vi "EV Loop Control.vi"(0 "Run Step Inputs":T1={"Data in"=[], "Results in"=[], "Seq Setup in"="", "Step name"="", "Hardware in"="", "Calibration in"="", "Step # in sequence"=0, "Display step?(f)"=TRUE, "Generate names only"=FALSE, "Waveforms in"=[], "Memory List Grouping info"=[]} {"Waveforms in"."Y dB ref" format="%.1f"; "Waveforms in"."Y axis" items=["dB", "Lin", "Pwr"]; "Waveforms in"."Y data" items=["dB", "Lin", "Pwr"]; "Waveforms in"."X data" items=["dB", "Lin", "Pwr"]; "Data in"."Z data" items=["dB", "Lin", "Pwr"]; "Data in"."X data" items=["dB", "Lin", "Pwr"]; "Data in"."Y data" items=["dB", "Lin", "Pwr"]; "Data in"."Z dB ref" format="%.1f"; "Data in"."Z axis" items=["Log", "Lin"]; "Data in"."X dB ref" format="%.1f"; "Data in"."X axis" items=["Log", "Lin"]; "Data in"."Y axis" items=["Log", "Lin"]; "Data in"."Y dB ref" format="%.1f"; "Data in"."Curve"."z" format="%.2f"; "Data in"."Curve"."y" format="%.2f"; "Data in"."Curve"."x" format="%.2f"; "Results in"."Unit type" items=["dB", "Lin", "Pwr"]; "Results in"."Margin" format="%.2f"}, 11 "error in (no error)":errorcluster) -> (6 "Data out":T2 {"Z data" items=["dB", "Lin", "Pwr"]; "X data" items=["dB", "Lin", "Pwr"]; "Y data" items=["dB", "Lin", "Pwr"]; "Z dB ref" format="%.1f"; "Z axis" items=["Log", "Lin"]; "X dB ref" format="%.1f"; "X axis" items=["Log", "Lin"]; "Y axis" items=["Log", "Lin"]; "Y dB ref" format="%.1f"; "Curve"."z" format="%.2f"; "Curve"."y" format="%.2f"; "Curve"."x" format="%.2f"}, 8 "Results out":T5 {"Unit type" items=["dB", "Lin", "Pwr"]; "Margin" format="%.2f"}, 10 "Waveforms out":T7 {"Y dB ref" format="%.1f"; "Y axis" items=["dB", "Lin", "Pwr"]; "Y data" items=["dB", "Lin", "Pwr"]; "X data" items=["dB", "Lin", "Pwr"]}, 15 "error out":errorcluster)   [LabVIEW 2014]
uses:
  custom and SC Run Seq Sub VIs (x64).llb/data array.ctl
  custom and SC Run Seq Sub VIs (x64).llb/data cluster.ctl
  custom and SC Run Seq Sub VIs (x64).llb/Axis Unit Type.ctl
  custom and SC Run Seq Sub VIs (x64).llb/result array.ctl
  custom and SC Run Seq Sub VIs (x64).llb/result cluster.ctl
  custom and SC Run Seq Sub VIs (x64).llb/waveform array.ctl
  custom and SC Run Seq Sub VIs (x64).llb/waveform cluster.ctl
  custom and SC Run Seq Sub VIs (x64).llb/Run Step Inputs.ctl
  custom and SC Run Seq Sub VIs (x64).llb/Memory List Grouping.ctl
  custom and SC Run Seq Sub VIs (x64).llb/Memory List Grouping - Item Type.ctl
  custom and SC Run Seq Sub VIs (x64).llb/window stack manager Functions.ctl
panel:
  out "mp curve":cluster{"x":dbl, "y":dbl, "z":dbl}[](array[cluster])
  out "inc curve":cluster{"x":dbl, "y":dbl, "z":dbl}[](array[cluster])
  out "x > 0?":bool
  out "size(s)":i32
  out "Numeric":dbl
  out "y":dbl
  out "x":dbl
  # "NOTE:  These controls and indicators must stay here, but you can Hide them if you wish.  These are wired as the standard input/output connector pane for step run VIs."
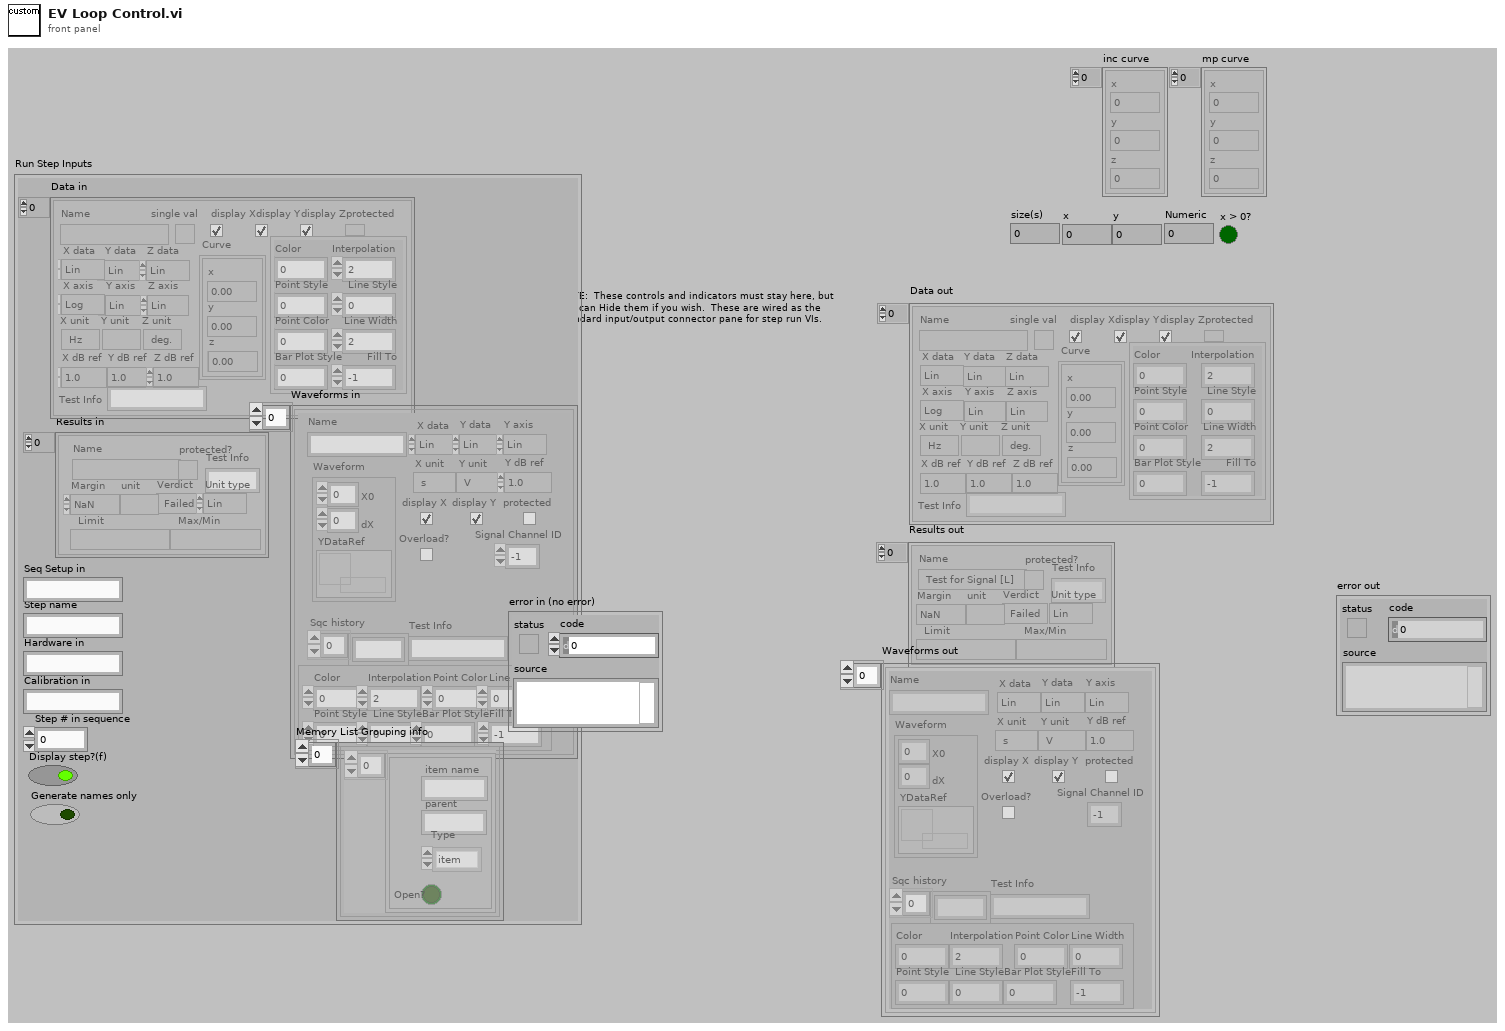
[diagram p1: front panel]
types:
  T1 = typedef "Run Step Inputs.ctl" = cluster{"Data in":T2, "Results in":T5, "Seq Setup in":string, "Step name":string, "Hardware in":string, "Calibration in":string, "Step # in sequence":i32, "Display step?(f)":bool, "Generate names only":bool, "Waveforms in":T7, "Memory List Grouping info":cluster{T9[]}[]}
  T2 = typedef "data array.ctl" = T3[]
  T3 = typedef "data cluster.ctl" = cluster{"Name":string, "Curve":cluster{"x":dbl, "y":dbl, "z":dbl}[], "X data":T4, "Y data":T4, "Z data":T4, "X axis":u16, "Y axis":u16, "Z axis":u16, "X unit":string, "Y unit":string, "Z unit":string, "X dB ref":dbl, "Y dB ref":dbl, "Z dB ref":dbl, "single val":bool, "protected":bool, "display X":bool, "display Y":bool, "display Z":bool, "Plot Settings":cluster{"Color":u32, "Interpolation":u8, "Point Style":u8, "Line Style":u8, "Point Color":u32, "Line Width":u8, "Bar Plot Style":u8, "Fill To":i16}, "Test Info":string}
  T4 = typedef "Axis Unit Type.ctl" = u16
  T5 = typedef "result array.ctl" = T6[]
  T6 = typedef "result cluster.ctl" = cluster{"Name":string, "Margin":dbl, "unit":string, "Verdict":bool, "Limit":string, "Max/Min":string, "protected?":bool, "Test Info":string, "Unit type":T4}
  T7 = typedef "waveform array.ctl" = T8[]
  T8 = typedef "waveform cluster.ctl" = cluster{"Name":string, "Waveform":cluster{"X0":dbl, "dX":dbl, "YDataRef":refnum<data-value>}, "X data":T4, "Y data":T4, "Y axis":T4, "X unit":string, "Y unit":string, "Y dB ref":dbl, "display Y":bool, "display X":bool, "Overload?":bool, "protected":bool, "Sqc history":string[], "Signal Channel ID":i32, "Plot Settings":cluster{"Color":u32, "Interpolation":u8, "Point Style":u8, "Line Style":u8, "Point Color":u32, "Line Width":u8, "Bar Plot Style":u8, "Fill To":i16}, "Test Info":string}
  T9 = typedef "Memory List Grouping.ctl" = cluster{"item name":string, "parent":string, "Open?":bool, "Type":T10}
  T10 = typedef "Memory List Grouping - Item Type.ctl" = enum16{"item", "custom group", "auto group", "protected group"}
  T11 = typedef "window stack manager Functions.ctl" = enum16{"Init", "add", "remove", "run", "clear", "vi stopped offset", "minimize all", "restore all", "autoadd", "Hourglass On", "Hourglass Off"}
  T12 = typedef "seq step setup.ctl" = cluster{"Input Signal Channels":i32[], "Output Signal Channels":i32[], "Curves selected":string[][], "Curves generated":string[], "Step setup flat":string, "Trigger Signal Channel":i32, "Curves Generated Assumptions":cluster{"seq-setup in":string, "Relevant subset of mem list Grouping":cluster{T9[]}[]}}
  T13 = cluster{"Curve[0]":cluster{"x":dbl, "y":dbl, "z":dbl}, "Curve[1]":cluster{"x":dbl, "y":dbl, "z":dbl}, "Curve[2]":cluster{"x":dbl, "y":dbl, "z":dbl}, "Curve[3]":cluster{"x":dbl, "y":dbl, "z":dbl}, "Curve[4]":cluster{"x":dbl, "y":dbl, "z":dbl}, "Curve[5]":cluster{"x":dbl, "y":dbl, "z":dbl}, "Curve[6]":cluster{"x":dbl, "y":dbl, "z":dbl}, "Curve[7]":cluster{"x":dbl, "y":dbl, "z":dbl}, "Curve[8]":cluster{"x":dbl, "y":dbl, "z":dbl}}
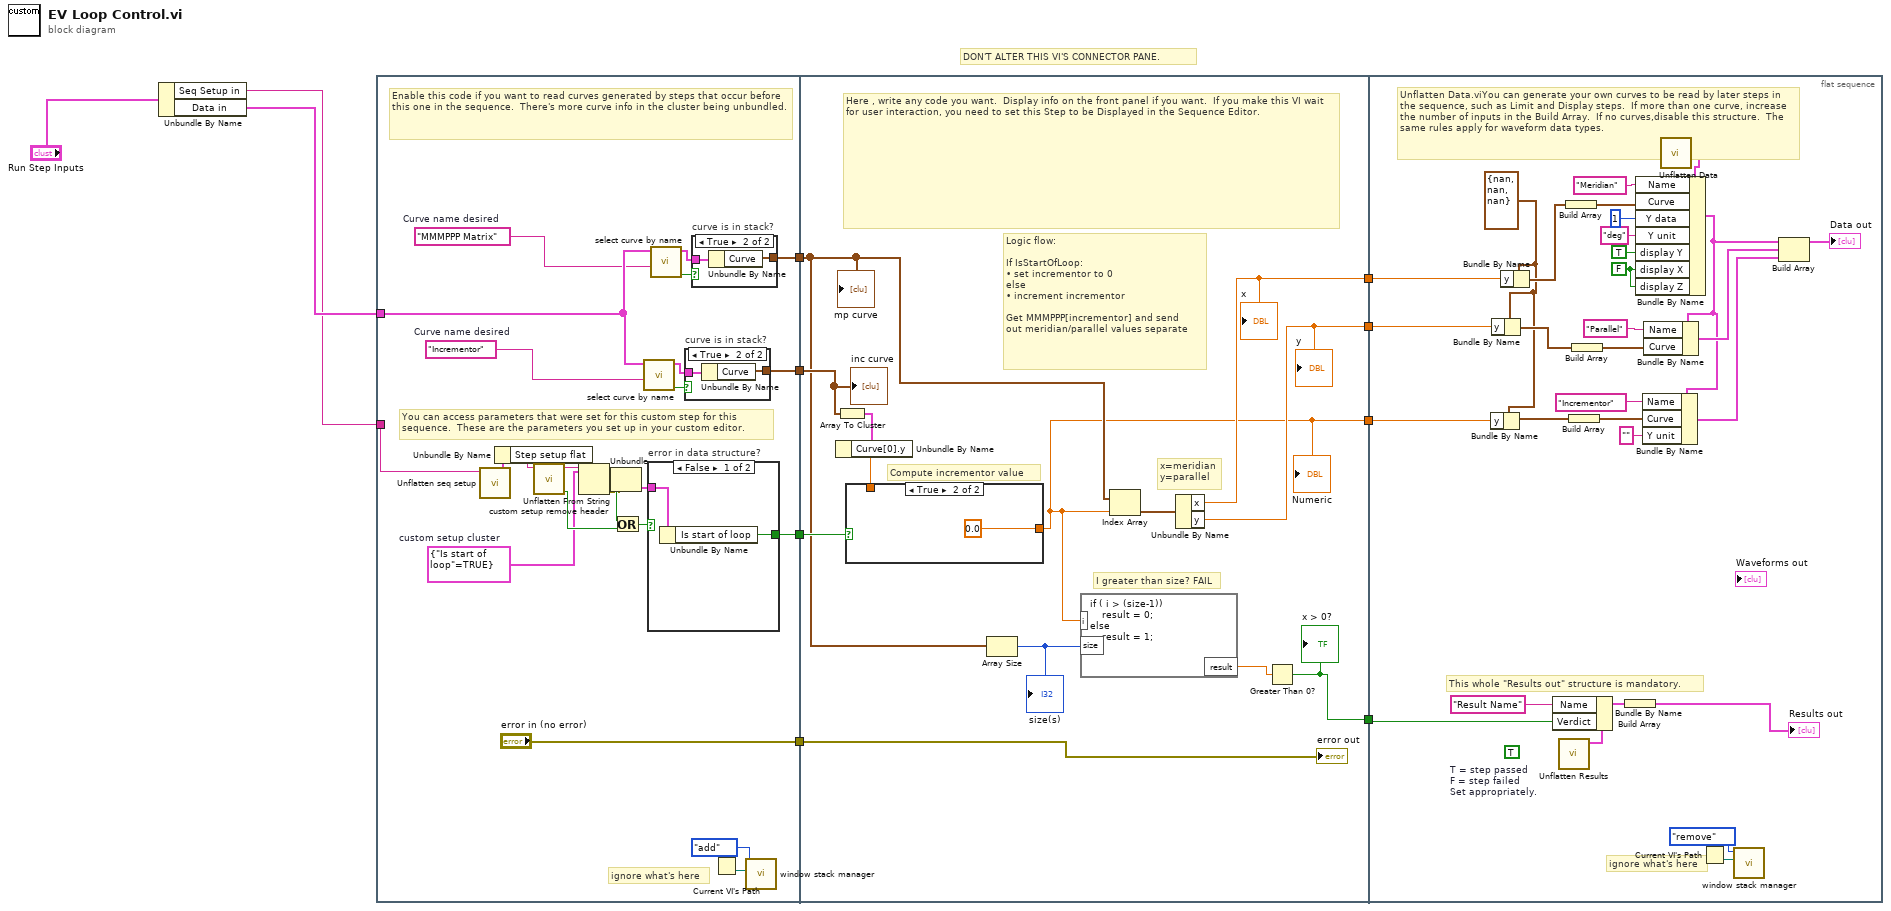
[diagram p0: block diagram]
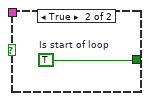
[diagram p4: hidden frame]
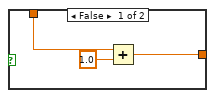
[diagram p5: hidden frame]
diagram:
  # "DON'T ALTER THIS VI'S CONNECTOR PANE."
  n1 = Unbundle By Name("Run Step Inputs") -> ("Seq Setup in"=w9:string, "Data in"=w10:T2)
  n2 = flat-sequence {
    tunnel: w10 -> [w15]
    tunnel: w9 -> [w25]
    tunnel: ["error in (no error)"] -> w8
    tunnel: [w19] -> w7
    tunnel: [w16] -> w6
    tunnel: [w14] -> w4
    tunnel: w8 -> [w54]
    tunnel: w7 -> [w53]
    tunnel: w6 -> [w52]
    tunnel: [w44] -> w5
    tunnel: w4 -> [w46]
    tunnel: [w48] -> w3
    tunnel: [w47] -> w2
    tunnel: [w42] -> w1
    tunnel: w5 -> [w79]
    tunnel: w3 -> [w78]
    tunnel: w2 -> [w77]
    tunnel: w1 -> [w71]
    frame #0 {
      w13 = "Incrementor"  # Curve name desired
      w12 = "MMMPPP Matrix"  # Curve name desired
      w22 = cluster{"Is start of loop":bool} {"Is start of loop"=TRUE}  # custom setup cluster
      # "ignore what's here"
      # "Enable this code if you want to read curves generated by steps that occur before this one in the sequence.  There's more curve info in the cluster being unbundled."
      # "You can access parameters that were set for this custom step for this sequence.  These are the parameters you set up in your custom editor."
      n3 = call "Unflatten seq setup.vi"("Unflatten seq setup"=w25) -> ("Sequence-specific step set-up"=w34:T12)  [unwired: 3 in, 7 out]
      n4 = Unbundle By Name(w34) -> ("Step setup flat"=w33:string)
      n5 = call "custom setup remove header.vi"("Output from 'Step setup flat' of seq-setup structure"=w33) -> ("Error?"=w31:bool, "Flattened custom step setup cluster"=w32:string)  [unwired: 9 out]
      n6 = Unflatten From String(type=w22, binary string=w32) -> (value=w28:cluster{"Is start of loop":bool}, error out=w27:errorcluster)  [unwired: 1 in, 3 out]
      n7 = Unbundle(w27) -> ("status"=w30:bool)  [unwired: 2 out]
      n8 = Or(x=w30, y=w31) -> (x .or. y?=w29:bool)
      n9 = call "select curve by name.vi"("Curve name desired (just name, if flat data not wired)"=w13, "Data array in"=w15) -> ("Exists?"=w18:bool, "Desired curve"=w17:T3)  [unwired: 1 in, 7 out]
      n10 = case "error in data structure?" shown="False" w29 {
        tunnel: [w40 w41] -> w19
        tunnel: w28 -> [w39 _]
        frame False {
          n11 = Unbundle By Name(w39) -> ("Is start of loop"=w40:bool)
        }
        frame True {
          w41 = TRUE  # Is start of loop
        }
      }
      n12 = call "select curve by name.vi"("Curve name desired (just name, if flat data not wired)"=w12, "Data array in"=w15) -> ("Exists?"=w21:bool, "Desired curve"=w20:T3)  [unwired: 1 in, 7 out]
      n13 = case "curve is in stack?" shown="True" w18 {
        tunnel: w17 -> [_ w36]
        tunnel: [_ w35] -> w16
        frame False {
        }
        frame True {
          n14 = Unbundle By Name(w36) -> ("Curve"=w35:cluster{"x":dbl, "y":dbl, "z":dbl}[])
        }
      }
      n15 = case "curve is in stack?" shown="True" w21 {
        tunnel: w20 -> [_ w38]
        tunnel: [_ w37] -> w14
        frame False {
        }
        frame True {
          n16 = Unbundle By Name(w38) -> ("Curve"=w37:cluster{"x":dbl, "y":dbl, "z":dbl}[])
        }
      }
      n17 = Current VI's Path() -> (path=w26:path)
      n18 = call "window stack manager.vi"("VI path"=w26, "Function (run)"=window_stack_manager_Functions."add") -> ()  [unwired: 5 in, 5 out]
    }
    frame #1 {
      # "I greater than size? FAIL"
      # "x=meridian\ny=parallel"
      # "Compute incrementor value"
      # "Logic flow:\n\nIf IsStartOfLoop:\n• set incrementor to 0\nelse\n• increment incrementor\n\nGet MMMPPP[incrementor] and send\nout meridian/parallel values separate"
      # "Here , write any code you want.  Display info on the front panel if you want.  If you make this VI wait for user interaction, you need to set this Step to be Displayed in the Sequence Editor."
      n19 = Array To Cluster(array=w52) -> (cluster=w51:T13)
      n20 = Unbundle By Name(w51) -> ("Curve[0].y"=w50:dbl)
      n21 = case shown="True" w53 {
        tunnel: [w55 0.0] -> w44
        tunnel: w50 -> [w57 _]
        frame False {
          n22 = Add(x=w57, y=1.0) -> (x+y=w55:dbl)
        }
        frame True {
        }
      }
      "Numeric" <- w44
      n23 = Array Size(array=w46) -> (size(s)=w45:i32)
      "size(s)" <- w45
      n24 = formula code="if ( i > (size-1))\n    result = 0;\nelse\n    result = 1;"("size"=w45, "i"=w44) -> ("result"=w43:dbl)
      n25 = Index Array(array=w46, index=w44) -> (element=w49:cluster{"x":dbl, "y":dbl, "z":dbl})
      n26 = Unbundle By Name(w49) -> ("x"=w48:dbl, "y"=w47:dbl)
      "x" <- w48
      "y" <- w47
      n27 = Greater Than 0?(x=w43) -> (x > 0?=w42:bool)
      "x > 0?" <- w42
      "error out" <- w54
      "inc curve" <- w52
      "mp curve" <- w46
    }
    frame #2 {
      w59 = FALSE ("display Y")
      w63 = cluster{"x":dbl, "y":dbl, "z":dbl} {"x"=nan, "y"=nan, "z"=nan}
      (unwired) TRUE  # T = step passed F = step failed Set appropriately.
      # "This whole \"Results out\" structure is mandatory."
      # "ignore what's here"
      # "Unflatten Data.viYou can generate your own curves to be read by later steps in the sequence, such as Limit and Display steps.  If more than one curve, increase the number of inputs in the Build Array.  If no curves,disable this structure.  The same rules apply for waveform data types."
      n28 = Bundle By Name(cluster=w63, "y"=w79) -> (w64:cluster{"x":dbl, "y":dbl, "z":dbl})
      n29 = Bundle By Name(cluster=w63, "y"=w77) -> (w66:cluster{"x":dbl, "y":dbl, "z":dbl})
      n30 = Bundle By Name(cluster=w63, "y"=w78) -> (w69:cluster{"x":dbl, "y":dbl, "z":dbl})
      n31 = call "Unflatten Results.vi"() -> ("Result"=w73:T6)  [unwired: 1 in, 10 out]
      n32 = Bundle By Name(cluster=w73, "Name"="Result Name", "Verdict"=w71) -> (w74:T6)
      n33 = Build Array(w69) -> (w68:cluster{"x":dbl, "y":dbl, "z":dbl}[])
      n34 = Build Array(w64) -> (w65:cluster{"x":dbl, "y":dbl, "z":dbl}[])
      n35 = Build Array(w66) -> (w67:cluster{"x":dbl, "y":dbl, "z":dbl}[])
      n36 = Build Array(w74) -> (→"Results out":T6[])
      n37 = call "Unflatten Data.vi"() -> ("Datum"=w76:T3)  [unwired: 1 in, 10 out]
      n38 = Bundle By Name(cluster=w76, "Name"="Meridian" ("Bundle Element"), "Curve"=w68, "Y data"=u16 1 ("0 = dB\n1 = linear"), "Y unit"="deg", "display Y"=TRUE ("display X"), "display X"=w59, "display Z"=w59) -> (w70:T3)
      n39 = Bundle By Name(cluster=w70, "Name"="Incrementor" ("Bundle Element"), "Curve"=w65, "Y unit"="") -> (w80:T3)
      n40 = Bundle By Name(cluster=w70, "Name"="Parallel" ("Bundle Element"), "Curve"=w67) -> (w82:T3)
      n41 = Current VI's Path() -> (path=w87:path)
      n42 = call "window stack manager.vi"("VI path"=w87, "Function (run)"=window_stack_manager_Functions."remove") -> ()  [unwired: 5 in, 5 out]
      n43 = Build Array(w70, w82, w80) -> (→"Data out":T3[])
    }
  }
